vi "Opencv_Image2Array.vi"(8 "error in (no error)":errorcluster, 11 "filename":string) -> (0 "error out":errorcluster, 2 "Image Pixels Gray":u8[][](array[numeric]), 3 "Image Pixels 24 bits":u32[][](array[numeric]))   [LabVIEW 2014, in "QwaveSys Raspberry Pi Library.lvlib"]
uses:
  QwaveSys Raspberry Pi Library.lvlib
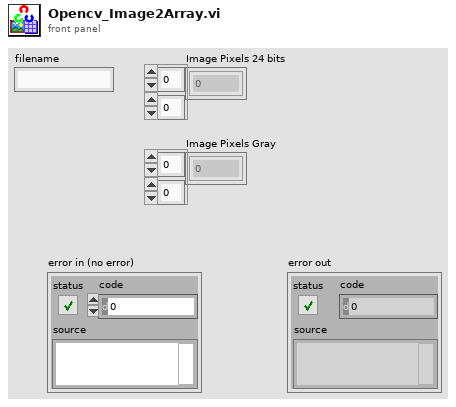
[diagram p1: front panel]
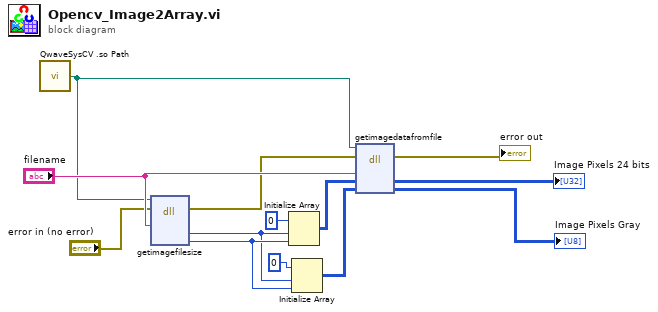
[diagram p0: block diagram]
diagram:
  n1 = call "QwaveSysCV .so Path.vi"() -> ("QwaveSys .so Path"=w4:path)  [unwired: 5 in]
  n2 = dll-call lib="libqwavesys.so" fn="getimagefilesize"(path in=w4, error in="error in (no error)", "filename"="filename") -> (error out=w3:errorcluster, "rows"=w10:i32, "cols"=w11:i32)  [unwired: 5 in, 1 out]
  n3 = Initialize Array(u32 0 ("element"), w10, w11) -> (w8:u32[][])
  n4 = Initialize Array(u8 0 ("element"), w10, w11) -> (w12:u8[][])
  n5 = dll-call lib="libqwavesys.so" fn="getimagedatafromfile"(path in=w4, error in=w3, "filename"="filename", "image"=w8, "gray"=w12) -> (error out=→"error out":errorcluster, "image"=→"Image Pixels 24 bits":u32[][], "gray"=→"Image Pixels Gray":u8[][])  [unwired: 3 in, 1 out]
